vi "Auto Drive Elev.vi"(0 "Left Side Speed":dbl, 2 "Right Side Speed":dbl, 5 "Elevator Height":dbl, 6 "Left Side Reset":bool, 7 "Right Side Reset":bool, 8 "Left Upper Limit":dbl, 9 "Right Upper Limit":dbl, 10 "Left Lower Limit":dbl, 11 "Right Lower Limit":dbl, 12 "Up Shift":bool, 13 "Down Shift":bool) -> (14 "Encoder Status":T1, 16 "Encoder Status 2":T1, 19 "Encoder Status 3":T1)   [LabVIEW 2014]
uses:
  <vilib>/Rock Robotics/WPI/RobotDrive/WPI_RobotDriveGetSetRefNum.vi
  <vilib>/Rock Robotics/Network Tables/SD Write Numeric Array.vi
  <vilib>/Rock Robotics/WPI/Solenoid/Deprecated/WPI_SolenoidSetBool.vi
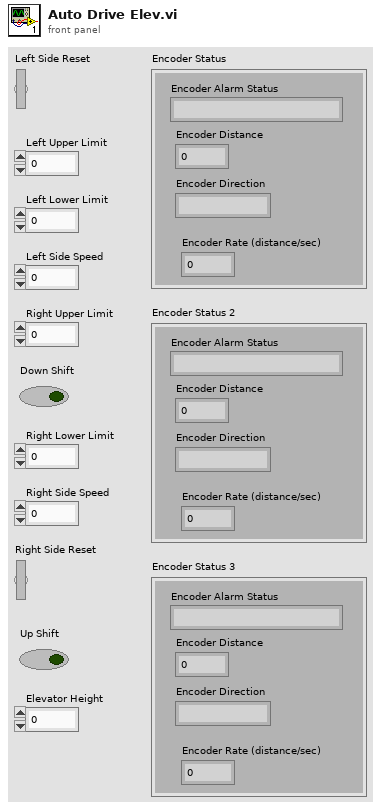
[diagram p1: front panel]
types:
  T1 = cluster{"Encoder Alarm Status":string, "Encoder Distance":dbl, "Encoder Direction":string, "Encoder Rate (distance/sec)":dbl}
  T2 = typedef "WPI_SolenoidDevRef.ctl" = cluster{"DevStatus":errorcluster, "Pneumatics Control Module":u8, "Forward Solenoid Channel":T3, "Reverse Solenoid Channel":T3}
  T3 = typedef "WPI_SolenoidChannel.ctl" = enum8{"Solenoid 0", "Solenoid 1", "Solenoid 2", "Solenoid 3", "Solenoid 4", "Solenoid 5", "Solenoid 6", "Solenoid 7", "Invalid"}
  T4 = cluster{"P Gain":dbl, "I Gain":dbl, "D Gain":dbl, "t":dbl}
  T5 = typedef "WPI_DigitalInputDevRef.ctl" = cluster{"DevStatus":errorcluster, "DIO Channel":T6, "Controller":T7}
  T6 = typedef "FPGA_DIOChannel.ctl" = enum8{"DIO 0", "DIO 1", "DIO 2", "DIO 3", "DIO 4", "DIO 5", "DIO 6", "DIO 7", "DIO 8", "DIO 9", "DIO MXP 0", "DIO MXP 1", "DIO MXP 2", "DIO MXP 3", "DIO MXP 4", "DIO MXP 5", "DIO MXP 6", "DIO MXP 7", "DIO MXP 8", "DIO MXP 9", "DIO MXP 10", "DIO MXP 11", "DIO MXP 12", "DIO MXP 13", "DIO MXP 14", "DIO MXP 15", "Invalid"}
  T7 = typedef "FPGA_TypedefDigitalModule.ctl" = enum16{"Controller 1"}
  T8 = cluster{"Elevator Height":dbl, "Output offset":dbl, "Value":bool}
  T9 = cluster{dbl, "Output offset":dbl, "Left Side Reset":bool}
  T10 = cluster{dbl, "Output offset":dbl, "Right Side Reset":bool}
  T11 = typedef "WPI_MotorControlDeviceRef.ctl" = cluster{"DeviceStatus":errorcluster, "Type":T12, "PWM":cluster{"Controller":T7, "PWM Channel":T13, "DeadBand":T14}, "CAN":cluster{"Device Number":u8, "Control Mode":T15, "Semaphore":T16, "Max Vout":dbl, "TalonSRX Control Mode":T17}, "Invert":bool, "TransformRef":T18, "InvTransformRef":T18}
  T12 = typedef "WPI_MotorControlType.ctl" = enum16{"PWM", "CAN", "CANTalonSRX"}
  T13 = typedef "FPGA_DIOPWMChannel.ctl" = enum8{"PWM 0", "PWM 1", "PWM 2", "PWM 3", "PWM 4", "PWM 5", "PWM 6", "PWM 7", "PWM 8", "PWM 9", "PWM MXP 0", "PWM MXP 1", "PWM MXP 2", "PWM MXP 3", "PWM MXP 4", "PWM MXP 5", "PWM MXP 6", "PWM MXP 7", "PWM MXP 8", "PWM MXP 9", "Invalid"}
  T14 = typedef "WPI_PWMDeadband.ctl" = cluster{"Name":string, "maxPositivePwm":i32, "minPositivePwm":i32, "centerPwm":i32, "maxNegativePwm":i32, "minNegativePwm":i32, "angularRange":u16}
  T15 = typedef "WPI_CANJaguar_ControlMode.ctl" = enum8{"Percent VBus", "Current", "Speed", "Position", "Voltage"}
  T16 = typedef "Semaphore RefNum" = refnum<k1>
  T17 = typedef "WPI_CANTalonSRX_APIControlMode.ctl" = enum8{"Percent VBus", "Speed", "Position", "Slave", "Unchanged / Invalid"}
  T18 = typedef "WPI_PWMTransform_ConPane.ctl" = refnum<vi>
  T19 = cluster{"Right Up Limit":dbl, "Right Lwr Limit":dbl}
  T20 = cluster{"Left Up Limit":dbl, "Left Lwr Limit":dbl}
  T21 = typedef "WPI_RobotDriveDevRef.ctl" = cluster{"DevStatus":errorcluster, "Motors[]":T11[], "Square Inputs":bool, "Max Output":dbl}
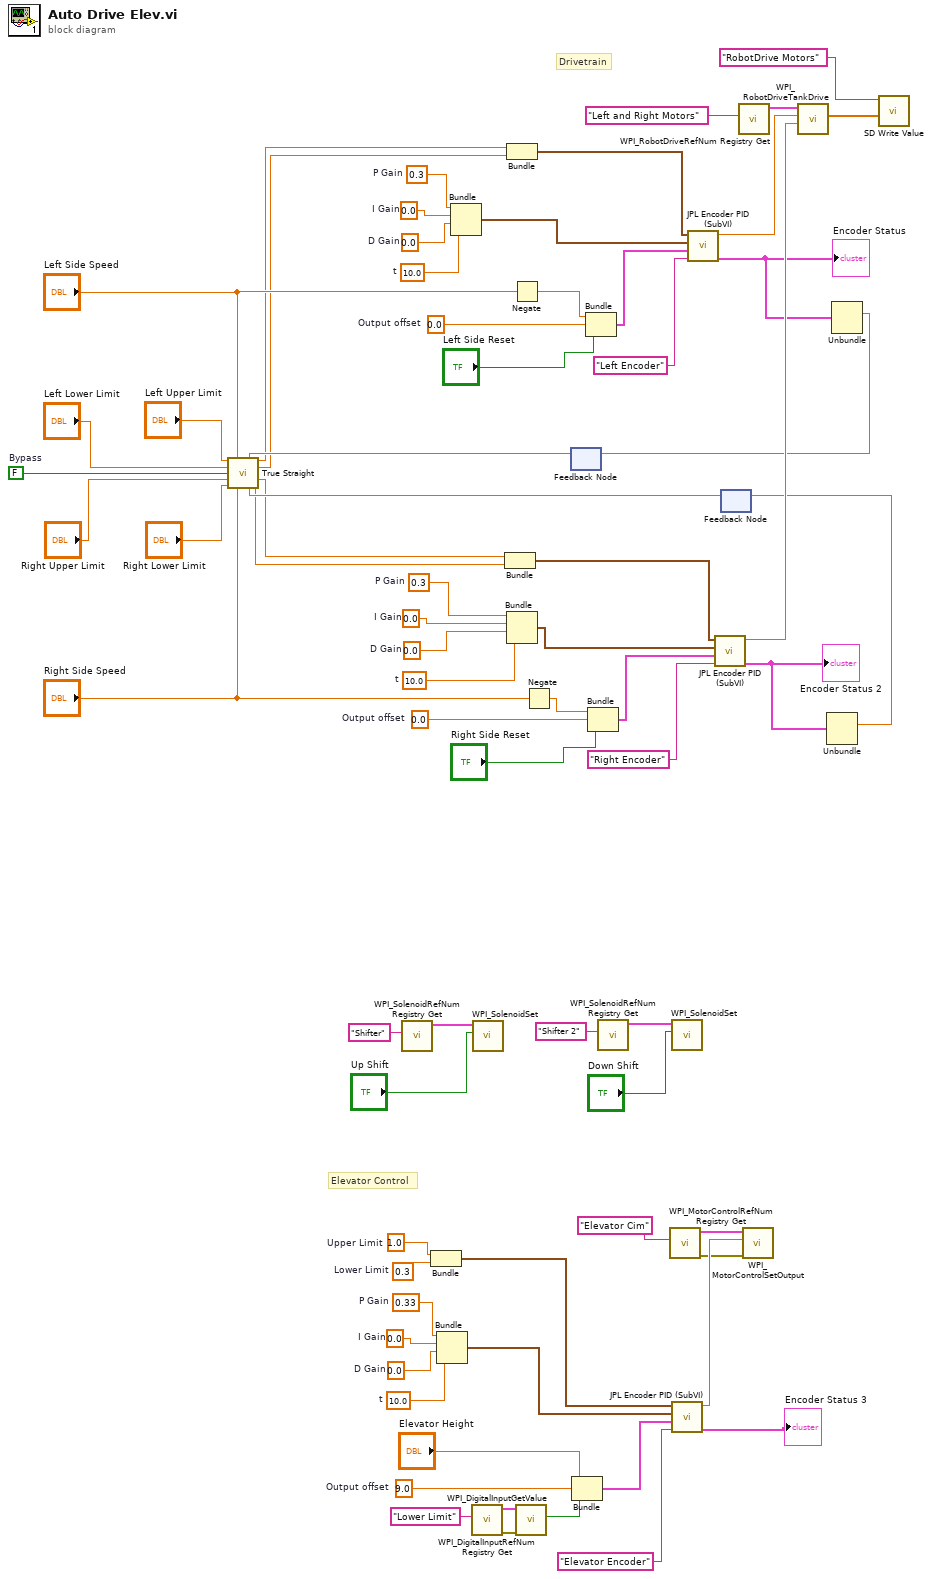
[diagram p0: block diagram]
diagram:
  w1 = FALSE  # Bypass
  w64 = 10.0  # t
  w63 = 0.0  # D Gain
  w62 = 0.0  # I Gain
  w61 = 0.3  # P Gain
  w60 = 0.0  # Output offset
  w55 = 10.0  # t
  w54 = 0.0  # D Gain
  w53 = 0.0  # I Gain
  w52 = 0.3  # P Gain
  w51 = 0.0  # Output offset
  w44 = 1.0  # Upper Limit
  w49 = 10.0  # t
  w48 = 0.0  # D Gain
  w47 = 0.0  # I Gain
  w46 = 0.33  # P Gain
  w43 = 0.3  # Lower Limit
  w40 = 9.0  # Output offset
  # "Elevator Control"
  # "Drivetrain"
  n1 = call <vilib>:"WPI_SolenoidRefNum Registry Get.vi"("refnum name"="Shifter") -> ("SolenoidDevRef"=w31:T2)  [unwired: 9 in, 1 out]
  n2 = Bundle("Upper Limit"=w44, "Lower Limit"=w43) -> (w71:cluster{"Upper Limit":dbl, "Lower Limit":dbl})  [unwired: 1 in]
  n3 = Bundle("P Gain"=w46, "I Gain"=w47, "D Gain"=w48, "t"=w49) -> (w45:T4)  [unwired: 1 in]
  n4 = Bundle("P Gain"=w52, "I Gain"=w53, "D Gain"=w54, "t"=w55) -> (w58:T4)  [unwired: 1 in]
  n5 = call <vilib>:"WPI_DigitalInputRefNum Registry Get.vi"("refnum name"="Lower Limit") -> ("error out"=w22:errorcluster, "DigitalInputDevRef"=w20:T5)  [unwired: 9 in]
  n6 = call-poly <vilib>:"WPI_SolenoidSet.vi"("Value"="Up Shift", "SolenoidDevRef"=w31) -> ()  [unwired: 8 in, 2 out]
  n7 = Bundle("P Gain"=w61, "I Gain"=w62, "D Gain"=w63, "t"=w64) -> (w67:T4)  [unwired: 1 in]
  n8 = Negate(x="Left Side Speed") -> (-x=w19:dbl)
  n9 = call <vilib>:"WPI_DigitalInputGetValue.vi"("error in (no error)"=w22, "DigitalInputDevRef"=w20) -> ("Value"=w39:bool)  [unwired: 7 in, 2 out]
  n10 = Negate(x="Right Side Speed") -> (-x=w18:dbl)
  n11 = feedback #1() -> (w11:dbl)  [unwired: 1 in]
  n12 = Bundle("Elevator Height"="Elevator Height", "Output offset"=w40, "Value"=w39) -> (w42:T8)  [unwired: 1 in]
  n13 = Bundle(w19, "Output offset"=w51, "Left Side Reset"="Left Side Reset") -> (w57:T9)  [unwired: 1 in]
  n14 = Bundle(w18, "Output offset"=w60, "Right Side Reset"="Right Side Reset") -> (w66:T10)  [unwired: 1 in]
  n15 = call <vilib>:"WPI_SolenoidRefNum Registry Get.vi"("refnum name"="Shifter 2") -> ("SolenoidDevRef"=w33:T2)  [unwired: 9 in, 1 out]
  n16 = call <vilib>:"WPI_MotorControlRefNum Registry Get.vi"("refnum name"="Elevator Cim") -> ("error out"=w24:errorcluster, "MotorControlDevRef"=w23:T11)  [unwired: 9 in]
  n17 = call-poly <vilib>:"WPI_SolenoidSet.vi"("Value"="Down Shift", "SolenoidDevRef"=w33) -> ()  [unwired: 8 in, 2 out]
  n18 = call "JPL Encoder PID (SubVI).vi"("refnum name"="Elevator Encoder", "Encoder Config"=w42, "PID Settings"=w45, "PID Limits"=w71) -> ("Encoder Status"=→"Encoder Status 3":T1, "output"=w50:dbl)  [unwired: 2 in]
  n19 = feedback #2() -> (w14:dbl)  [unwired: 1 in]
  n20 = call "True Straight.vi"("Left Upper Limit"="Left Upper Limit", "Left Speed"="Left Side Speed", "Left Encoder"=w11, "Left Lower Limit"="Left Lower Limit", "Bypass"=w1, "Right Upper Limit"="Right Upper Limit", "Right Lower Limit"="Right Lower Limit", "Right Speed"="Right Side Speed", "Right Encoder 2"=w14) -> ("Left Up Limit"=w5:dbl, "Left Lwr Limit"=w4:dbl, "Right Up Limit"=w3:dbl, "Right Lwr Limit"=w2:dbl)  [unwired: 3 in]
  n21 = Bundle("Right Up Limit"=w3, "Right Lwr Limit"=w2) -> (w68:T19)  [unwired: 1 in]
  n22 = Bundle("Left Up Limit"=w5, "Left Lwr Limit"=w4) -> (w59:T20)  [unwired: 1 in]
  n23 = call "JPL Encoder PID (SubVI).vi"("refnum name"="Left Encoder", "Encoder Config"=w57, "PID Settings"=w58, "PID Limits"=w59) -> ("Encoder Status"=w16:T1, "output"=w37:dbl)  [unwired: 2 in]
  "Encoder Status" <- w16
  n24 = call "JPL Encoder PID (SubVI).vi"("refnum name"="Right Encoder", "Encoder Config"=w66, "PID Settings"=w67, "PID Limits"=w68) -> ("Encoder Status"=w17:T1, "output"=w38:dbl)  [unwired: 2 in]
  "Encoder Status 2" <- w17
  n25 = call <vilib>:"WPI_RobotDriveRefNum Registry Get.vi"("refnum name"="Left and Right Motors") -> ("RobotDriveDevRef"=w28:T21)  [unwired: 1 in, 9 out]
  n26 = call <vilib>:"WPI_MotorControlSetOutput.vi"("error in (no error)"=w24, "Output"=w50, "MotorControlDevRef"=w23) -> ()  [unwired: 6 in, 3 out]
  n27 = call <vilib>:"WPI_RobotDriveTankDrive.vi"("Right axis value"=w38, "Left axis value"=w37, "RobotDriveDevRef"=w28) -> ("Motor Values"=w29:dbl[])  [unwired: 6 in, 2 out]
  n28 = Unbundle(w17) -> ("Encoder Distance"=w15:dbl)  [unwired: 3 out]
  n29 = feedback-in #2(w15) -> ()
  n30 = Unbundle(w16) -> ("Encoder Distance"=w12:dbl)  [unwired: 3 out]
  n31 = feedback-in #1(w12) -> ()
  n32 = call-poly <vilib>:"SD Write Value.vi"("Numeric Array"=w29, "Name"="RobotDrive Motors") -> ()  [unwired: 8 in, 2 out]
